vi "EuniceF_Project1Labview.vi"() -> ()   [LabVIEW 2025]
panel:
  out "Numeric":dbl format="%1.1g"
  out "A to D":i16 format="%x"
  in  "stop":bool
  out "LOW":bool
  out "GOOD":bool
  out "HIGH":bool
  out "Relative Humidity %":dbl(slide) scale=0.0..100.0
  out "Rsens, kOhms":dbl(slide) scale=20.0..40.0 scale format="%#_6f"
  out "V+,V":dbl(slide) scale=2.0..3.5
  out "Vdiff,V":dbl(slide) scale=-0.1..0.5
  out "VSS_C, V":dbl(slide) scale=-7.5..7.5 scale format="%0#1.4f"
  # "Technical Items"
  # "User Interface"
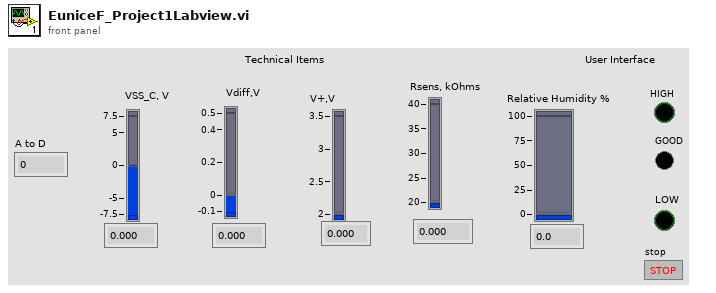
[diagram p1: front panel]
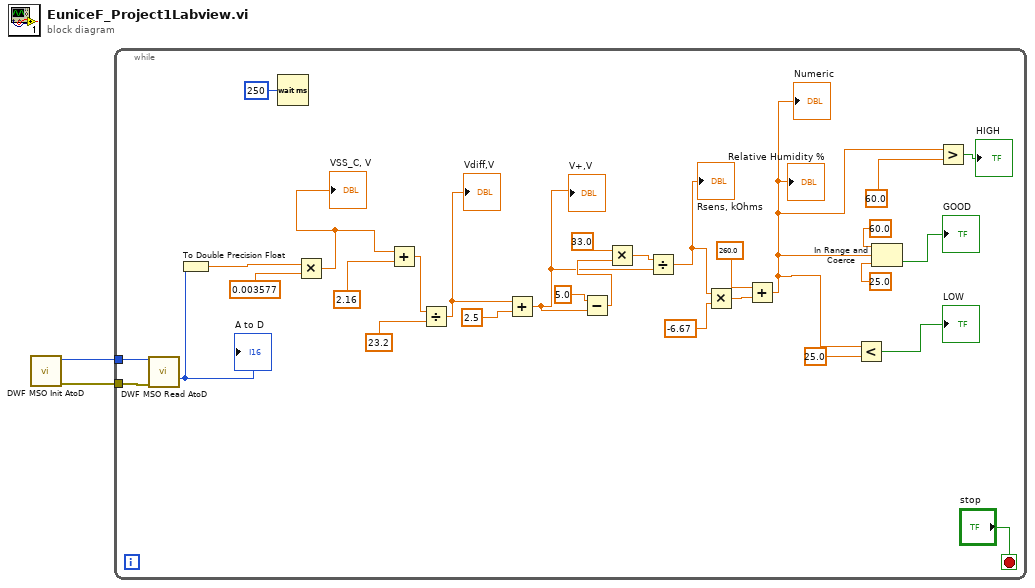
[diagram p0: block diagram]
diagram:
  n1 = call "DWF MSO Init AtoD.vi"() -> ("Error Out"=w2:errorcluster, "Instrument Handle Out"=w1:i32)  [unwired: 10 in]
  n2 = while {
    tunnel: w2 -> [w30]
    tunnel: w1 -> [w29]
    stop <- "stop" stop-if-true
    n3 = call "DWF MSO Read AtoD.vi"("Instrument Handle In AtoD"=w29, "Error In"=w30) -> ("AtoD"=w28:i16)  [unwired: 12 in, 1 out]
    "A to D" <- w28
    n4 = To Double Precision Float(number=w28) -> (double precision float=w23:dbl)
    n5 = Wait (ms)(milliseconds to wait=u32 250) -> ()  [unwired: 1 out]
    n6 = Multiply(x=w23, y=0.003577 ("x/y")) -> (x*y=w22:dbl)
    "VSS_C, V" <- w22
    n7 = Add(x=w22, y=2.16) -> (x+y=w24:dbl)
    n8 = Divide(x=w24, y=23.2) -> (x/y=w20:dbl)
    "Vdiff,V" <- w20
    n9 = Add(x=w20, y=2.5) -> (x+y=w3:dbl)
    "V+,V" <- w3
    n10 = Subtract(x=5.0 ("y"), y=w3) -> (x-y=w4:dbl)
    n11 = Multiply(x=33.0, y=w4) -> (x*y=w18:dbl)
    n12 = Divide(x=w18, y=w3) -> (x/y=w16:dbl)
    "Rsens, kOhms" <- w16
    n13 = Multiply(x=w16, y=-6.67) -> (x*y=w14:dbl)
    n14 = Add(x=260.0, y=w14) -> (x+y=w6:dbl)
    "Relative Humidity %" <- w6
    "Numeric" <- w6
    n15 = Less?(x=w6, y=25.0) -> (x < y?=→"LOW":bool)
    n16 = In Range and Coerce(upper limit=60.0, x=w6, lower limit=25.0) -> (In Range?=→"GOOD":bool)  [unwired: 1 out]
    n17 = Greater?(x=w6, y=60.0) -> (0:→"HIGH":bool)
  }
